vi "显示测试结果-左下角-显示图像处理信息.vi"(6 "每个数据结果":bool[](array[boolean]), 8 "显示坐标":cluster{dbl, "Numeric":dbl}[](array[cluster])=[{100.0, "Numeric"=1700.0}, {100.0, "Numeric"=1780.0}, {100.0, "Numeric"=1860.0}, {100.0, "Numeric"=1940.0}, {100.0, "Numeric"=2020.0}, {100.0, "Numeric"=2200.0}, {100.0, "Numeric"=2300.0}, {100.0, "Numeric"=2400.0}, {100.0, "Numeric"=2500.0}], 9 "量测项目名称":string[](array[string]), 10 "显示数据":dbl[](array[numeric]), 11 "Img输入":T1) -> ()   [LabVIEW 2014]
uses:
  <vilib>/vision/Image Controls.llb/IMAQ Image.ctl
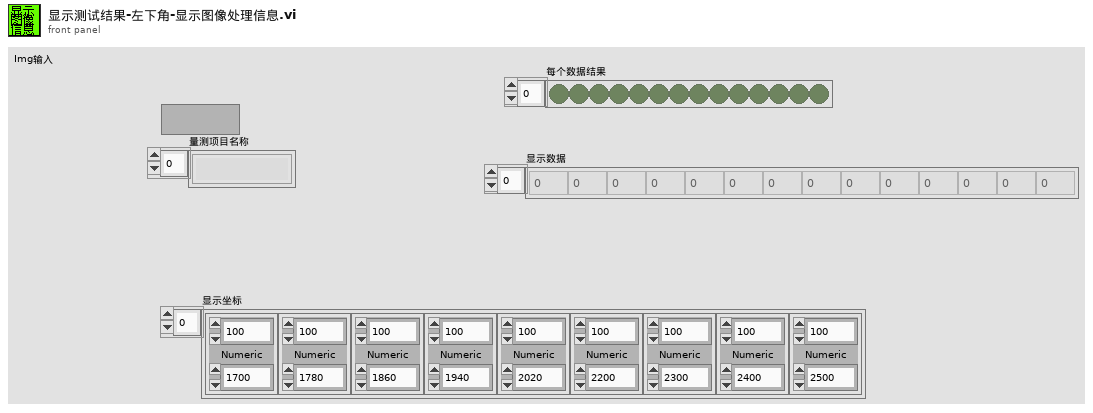
[diagram p1: front panel]
types:
  T1 = typedef "IMAQ Image.ctl" = refnum<image>
  T2 = cluster{"Desired Font (Application)":enum16{"User-specified Font", "Application Font", "System Font", "Dialog Font"}, "[User-specified Font]":cluster{"Font Name":string, "Size":i16, "Strikeout?":bool, "Italic?":bool, "Underline?":bool, "Outline?":bool, "Shadow?":bool, "Bold?":bool, "Rotation Angle":dbl}, "Horizontal Alignment":i16, "Vertical Alignment":i16}
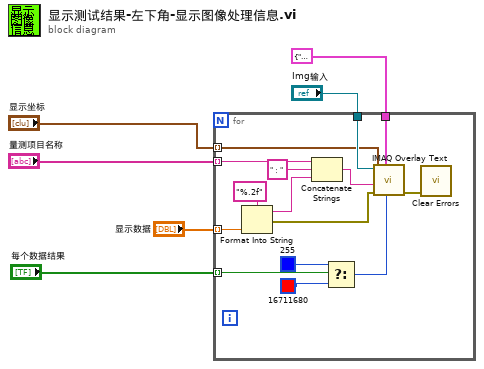
[diagram p0: block diagram]
diagram:
  n1 = for {
    tunnel: "Img输入" -> [w21]
    tunnel: "显示数据" -> [w20] mode=indexing
    tunnel: "显示坐标" -> [w19] mode=indexing
    tunnel: T2 {"Desired Font (Application)"=enum."User-specified Font", "[User-specified Font]"={"Font Name"="", "Size"=60, "Strikeout?"=FALSE, "Italic?"=FALSE, "Underline?"=FALSE, "Outline?"=FALSE, "Shadow?"=FALSE, "Bold?"=FALSE, "Rotation Angle"=0.0}, "Horizontal Alignment"=0, "Vertical Alignment"=0} ("Font, Size & Style") -> [w18]
    tunnel: "量测项目名称" -> [w14] mode=indexing
    tunnel: "每个数据结果" -> [w10] mode=indexing
    n2 = Format Into String(format string="%.2f" ("格式字符串"), w20) -> (resulting string=w12:string, error out=w16:errorcluster)  [unwired: 2 in]
    n3 = Concatenate Strings(w14, "：" ("字符串"), w12) -> (w13:string)
    n4 = Select(t=u32 255 ("Text Color (black)"), s=w10, f=u32 16711680 ("Text Color (black)")) -> (s? t:f=w7:u32)
    n5 = call "IMAQ Overlay Text"("Text Color (black)"=w7, "Font, Size & Style"=w18, "error in (no error)"=w16, "String"=w13, "Origin"=w19, "Image"=w21) -> ("error out"=w15:errorcluster)  [unwired: 4 in, 1 out]
    n6 = call <vilib>:"Clear Errors.vi"("error in (no error)"=w15) -> ()  [unwired: 5 in, 2 out]
  }
